vi "Stop Core.vi"(10 "final error code":i32, 11 "IViewable in":refnum<class "IViewable.lvclass">) -> (3 "IViewable out":refnum<class "IViewable.lvclass">)   [LabVIEW 2015, in "IViewable.lvlib" / "IViewable.lvclass"]
doc: "(<B>Filename</B>: Actor Framework.lvlib:Actor.lvclass:Stop Core.vi)\n\nDefines what the actor does before it stops. Use the <B>final error code</B> input to determine whether the actor shut down in response to an error.\n\nBy default, this method does nothing. A descendant class may override it to define behavior, such as shutting down any processes the actor initiated in its override of the Actor Core method."
uses:
  IViewable.lvclass
  IViewable.lvclass/IViewable.ctl
  AutoRegistration/AutoEventActor/AutoEventActor.lvclass
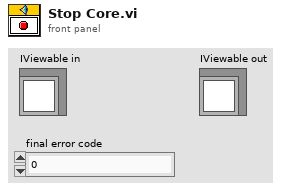
[diagram p1: front panel]
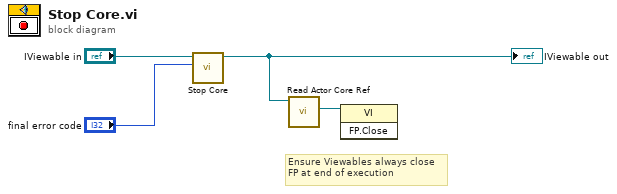
[diagram p0: block diagram]
diagram:
  # "Ensure Viewables always close\nFP at end of execution"
  n1 = call-parent "Stop Core.vi"("final error code"="final error code", "Actor in"="IViewable in") -> ("Actor out"=w2:refnum<class "IViewable.lvclass">)  [unwired: 9 in]
  "IViewable out" <- w2
  n2 = call "Read Actor Core Ref.vi"("IViewable In"=w2) -> ("Actor Core Ref"=w1:refnum<vi>)  [unwired: 8 in, 2 out]
  n3 = invoke class="VI" method="FP.Close"(reference=w1) -> ()  [unwired: 2 in, 3 out]
